vi "IO Channel Name Collision Check.vi"() -> (0 "Channel Names Collide":bool)   [LabVIEW 2013]
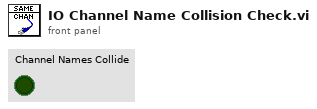
[diagram p1: front panel]
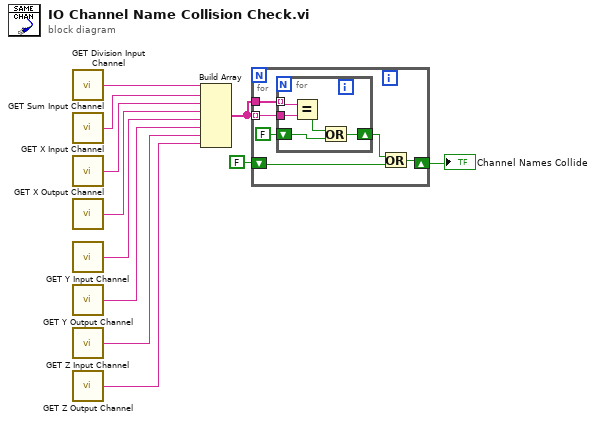
[diagram p0: block diagram]
diagram:
  n1 = call "GET Division Input Channel.vi"() -> ("Division Input Channel"=w11:string)
  n2 = call "GET Sum Input Channel.vi"() -> ("Sum Input Channel"=w10:string)
  n3 = call "GET X Input Channel.vi"() -> ("X Input Channel"=w9:string)
  n4 = call "GET X Output Channel.vi"() -> ("X Output Channel"=w8:string)
  n5 = call "GET Y Input Channel.vi"() -> ("Y Input Channel"=w7:string)
  n6 = call "GET Y Output Channel.vi"() -> ("Y Output Channel"=w6:string)
  n7 = call "GET Z Input Channel.vi"() -> ("Z Input Channel"=w5:string)
  n8 = call "GET Z Output Channel.vi"() -> ("Z Output Channel"=w4:string)
  n9 = Build Array(w11, w10, w9, w8, w7, w6, w5, w4) -> (w3:string[])
  n10 = for {
    tunnel: w3 -> [w16] mode=indexing
    tunnel: w3 -> [w17]
    shift-right: [w13] -> w1
    shift-left: FALSE -> [w12]
    n11 = for {
      tunnel: w17 -> [w21] mode=indexing
      tunnel: w16 -> [w22]
      shift-right: [w20] -> w14
      shift-left: FALSE -> [w18]
      n12 = Equal?(x=w21, y=w22) -> (x = y?=w19:bool)
      n13 = Or(x=w19, y=w18) -> (x .or. y?=w20:bool)
    }
    n14 = Or(x=w14, y=w12) -> (x .or. y?=w13:bool)
  }
  "Channel Names Collide" <- w1
